vi "ICsimpleTest.vi"() -> ()   [LabVIEW 2015]
panel:
  out "element":string
  out "Devices":string[](array[string])
  out "Error Out":errorcluster
  in  "Grab":bool
  in  "stop":bool
  in  "ICImagingControl":refnum<k7>(container)
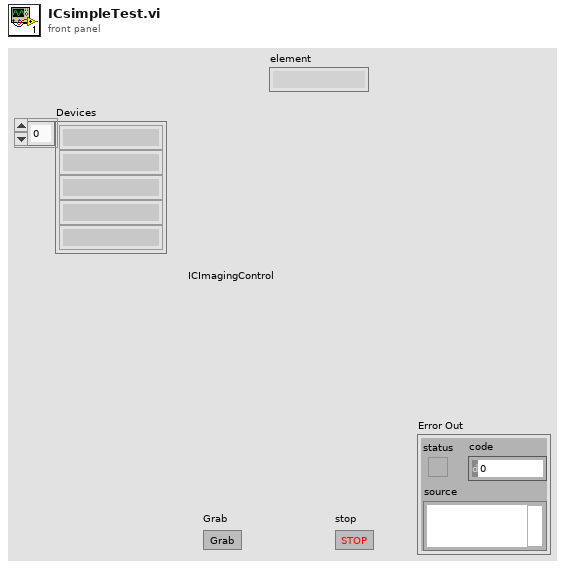
[diagram p1: front panel]
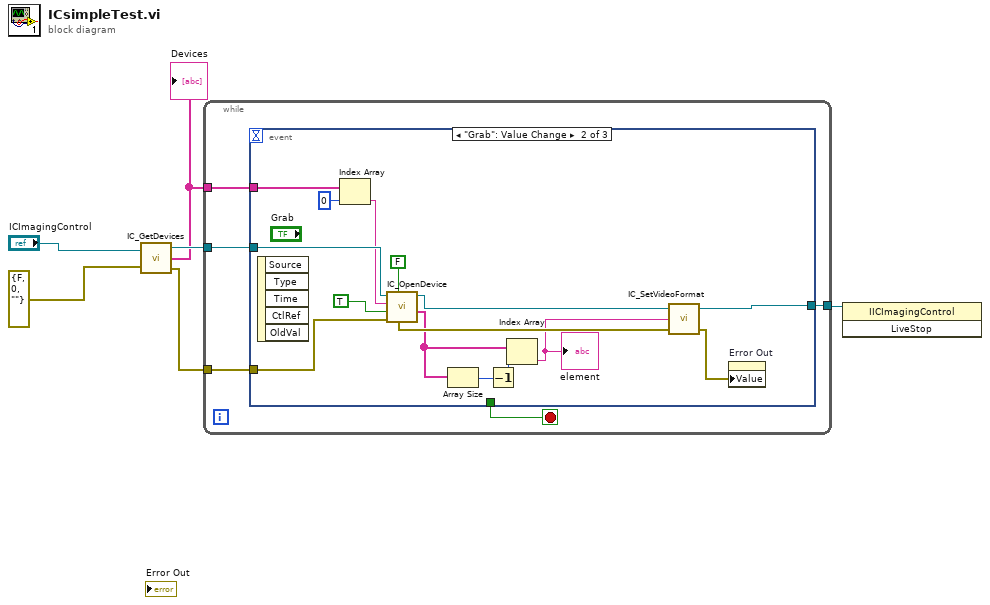
[diagram p0: block diagram]
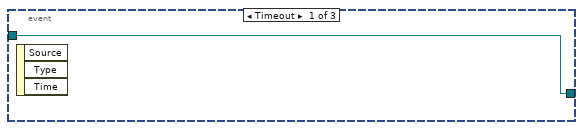
[diagram p2: hidden frame]
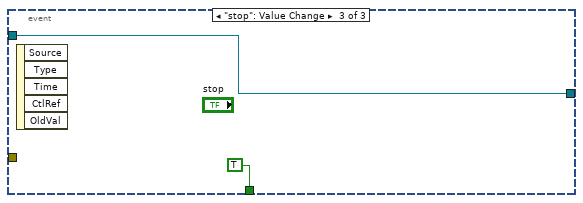
[diagram p3: hidden frame]
diagram:
  n1 = call <userlib>:"IC_GetDevices.vi"("ICImagingControl In"="ICImagingControl", "Error In (no error)"=errorcluster {"status"=FALSE, "code"=0, "source"=""}) -> ("ICImagingControl Out"=w3:refnum<k7>, "Devices"=w2:string[], "Error Out"=w4:errorcluster)
  "Devices" <- w2
  n2 = while {
    tunnel: w4 -> [w10]
    tunnel: w3 -> [w9]
    tunnel: w2 -> [w8]
    tunnel: [w7] -> w1
    stop <- w11 stop-if-true
    n3 = event shown="[1] \"Grab\": Value Change" {
      selector: _ -> [_ _ _]
      dyn-events: _ -> [_ _ _]
      timeout: _ -> [_ _ _]
      tunnel: [_ _ TRUE] -> w11
      tunnel: w10 -> [_ w27 _]
      tunnel: w9 -> [w12 w26 w28]
      tunnel: w8 -> [_ w25 _]
      tunnel: [w12 w13 w28] -> w7
      event Timeout {
        n4 = event-data() -> ()  [unwired: 1 in, 3 out]
      }
      event "Grab": Value Change {
        n5 = event-data() -> ()  [unwired: 1 in, 5 out]
        n6 = Index Array(array=w25, index=0) -> (element=w23:string)
        n7 = call <userlib>:"IC_OpenDevice.vi"("Color"=FALSE, "Error In (no error)"=w27, "Live"=TRUE, "Device"=w23, "ICImagingControl In"=w26) -> ("VideoFormats"=w19:string[], "ICImagingControl Out"=w15:refnum<k7>, "Error Out"=w21:errorcluster)  [unwired: 1 in, 3 out]
        n8 = Array Size(array=w19) -> (size(s)=w18:i32)
        n9 = Decrement(x=w18) -> (x-1=w17:i32)
        n10 = Index Array(array=w19, index=w17) -> (element=w16:string)
        "element" <- w16
        n11 = call <userlib>:"IC_SetVideoFormat.vi"("Error In (no error)"=w21, "VideoFormat"=w16, "ICImagingControl In"=w15) -> ("Error Out"=w20:errorcluster, "ICImagingControl Out"=w13:refnum<k7>)  [unwired: 1 out]
        n12 = property on="Error Out" class="Clust (strict)"("Value"=w20) -> ()  [unwired: 2 in, 2 out]
      }
      event "stop": Value Change {
        n13 = event-data() -> ()  [unwired: 1 in, 5 out]
      }
    }
  }
  n14 = invoke class="IICImagingControl" method="LiveStop"(reference=w1) -> ()  [unwired: 2 in, 3 out]
